vi "algorithm_4.2.vi"(10 "String":string) -> (2 "Score":i32)   [LabVIEW 2017]
uses:
  BingoBoard/BingoBoard.lvclass
panel:
  out "Numeric":i32
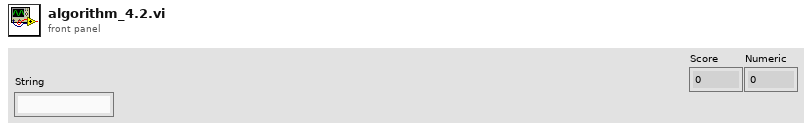
[diagram p1: front panel]
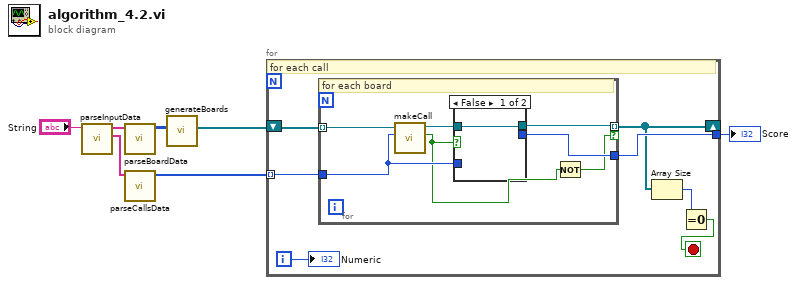
[diagram p0: block diagram]
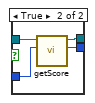
[diagram p2: hidden frame]
diagram:
  n1 = call "parseInputData.vi"("String"="String") -> ("CallsData"=w6:string[], "BoardsData"=w5:string[])  [unwired: 9 in]
  n2 = call "parseBoardData.vi"("Array in"=w5) -> ("Array out"=w4:i32[][][])  [unwired: 10 in]
  n3 = call "parseCallsData.vi"("Array in"=w6) -> ("Array out"=w3:i32[])  [unwired: 10 in]
  n4 = call "generateBoards.vi"("Array"=w4) -> ("BingoBoards"=w2:refnum<class "BingoBoard.lvclass">[])  [unwired: 10 in]
  n5 = for {
    tunnel: w3 -> [w13] mode=indexing
    tunnel: [w12] -> w1
    shift-right: [w10] -> _
    shift-left: w2 -> [w14]
    i -> [w11]
    stop <- w8 stop-if-true
    # "for each call"
    n6 = for {
      tunnel: w14 -> [w21] mode=indexing
      tunnel: w13 -> [w17]
      tunnel: [w19] -> w12
      tunnel: [w18] -> w10 mode=indexing if=w15
      # "for each board"
      n7 = call-dynamic "makeCall.vi"("call"=w17, "BingoBoard in"=w21) -> ("won?"=w16:bool, "BingoBoard out"=w20:refnum<class "BingoBoard.lvclass">)  [unwired: 7 in, 1 out]
      n8 = case shown="False" w16 {
        tunnel: w20 -> [w22 w26]
        tunnel: [_ w25] -> w19
        tunnel: [w22 w24] -> w18
        tunnel: w17 -> [_ w23]
        frame False {
        }
        frame True {
          n9 = call-dynamic "getScore.vi"("call"=w23, "BingoBoard in"=w26) -> ("Score"=w25:i32, "BingoBoard out"=w24:refnum<class "BingoBoard.lvclass">)  [unwired: 7 in, 1 out]
        }
      }
      n10 = Not(x=w16) -> (.not. x?=w15:bool)
    }
    n11 = Array Size(array=w10) -> (size(s)=w9:i32)
    n12 = Equal To 0?(x=w9) -> (x = 0?=w8:bool)
    "Numeric" <- w11
  }
  "Score" <- w1
